vi "Call Chain To Indent.vi"(11 "Call Chain":string[](array[string])) -> (3 "Indent":string)   [LabVIEW 2009, in "Caraya.lvlib" / "Basic Test Manager.lvclass"]
uses:
  Basic Test Manager.lvclass
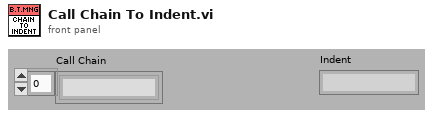
[diagram p1: front panel]
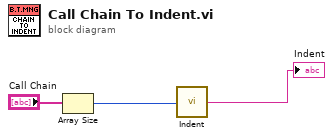
[diagram p0: block diagram]
diagram:
  n1 = Array Size(array="Call Chain") -> (size(s)=w3:i32)
  n2 = call "Indent.vi"("Numeric"=w3) -> ("string"=→"Indent":string)
